vi "Update Test Parameter.vi"(8 "error in (no error)":errorcluster) -> (0 "error out":errorcluster)   [LabVIEW 2016, in "User Interface.lvlib"]
uses:
  User Interface.lvlib
  Test Status Command.ctl
panel:
  in  "Unit":string
  in  "result":bool
  in  "Actual":string
  in  "LSL":string
  in  "USL":string
  in  "Control Ref.Test Result":refnum<vi>
  in  "Test Case ID":i32
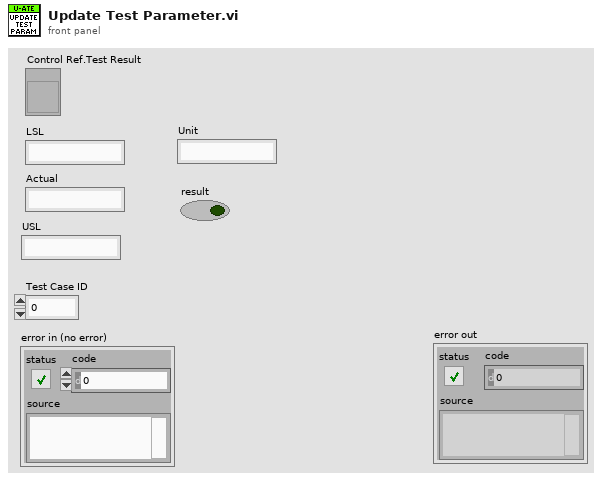
[diagram p1: front panel]
types:
  T1 = typedef "User Interface.lvlib/Test Status Command.ctl" = enum16{"Init", "Test Status"}
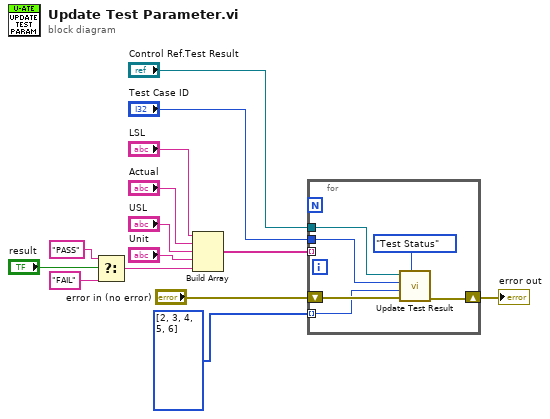
[diagram p0: block diagram]
diagram:
  n1 = Select(t="PASS", s="result", f="FAIL") -> (s? t:f=w10:string)
  n2 = Build Array("LSL", "Actual", "USL", "Unit", w10) -> (w4:string[])
  n3 = for {
    tunnel: "Control Ref.Test Result" -> [w18]
    tunnel: "Test Case ID" -> [w16]
    shift-right: [w19] -> w5
    shift-left: "error in (no error)" -> [w20]
    tunnel: w4 -> [_] mode=indexing
    tunnel: i32[] [2, 3, 4, 5, 6] -> [w15] mode=indexing
    n4 = call "Update Test Result.vi"("Command"=Test_Status_Command."Test Status", "error in (no error)"=w20, "Table Index"=w15, "Test ID Index"=w16, "Test Result"=w18) -> ("error out"=w19:errorcluster)  [unwired: 6 in]
  }
  "error out" <- w5
